vi "Handler - Fast Acq Loop.vi"(7 "Acquisition Start?":bool, 8 "error in (no error)":errorcluster, 9 "Acq Loop Data":T1, 10 "Loop Period":i64, 11 "Acquisition Period":i64) -> (0 "error out":errorcluster)   [LabVIEW 2018]
uses:
  Variables/Global - Data Globals.vi
  <vilib>/ptbypt/NI_PtbyPt.lvlib
  FPGA/Controls/DAQ Input Data.ctl
  Private Controls/FPGA Write Queue Data.ctl
  Outputs.lvlib
  Private Controls/Acquisition Loop Data.ctl
  FPGA/FPGA VI Reference.ctl
  <vilib>/Modbus/master/Modbus Master.lvclass
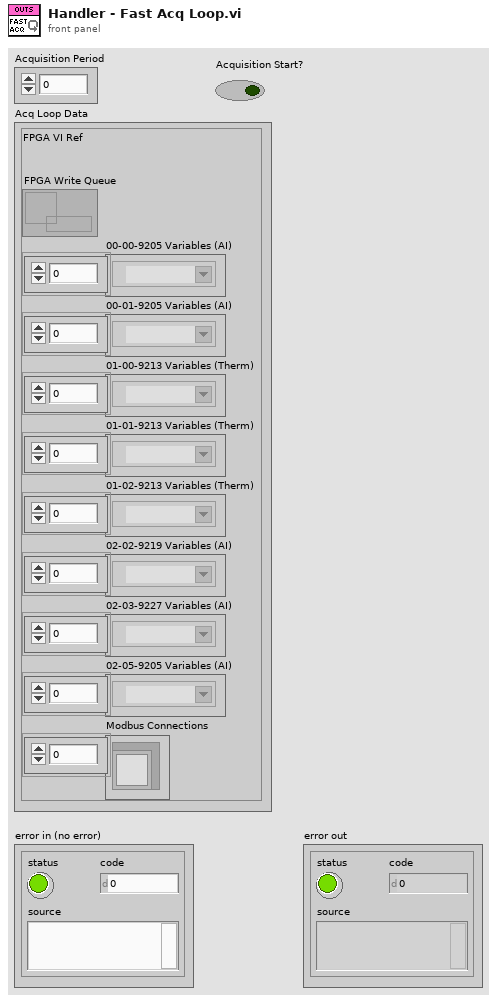
[diagram p1: front panel]
types:
  T1 = typedef "RT - Instrument IO.lvlib/Acquisition Loop Data.ctl" = cluster{"FPGA VI Ref":T2, "FPGA Write Queue":refnum<queue>, "00-00-9205 Variables (AI)":refnum<k21>[], "00-01-9205 Variables (AI)":refnum<k21>[], "01-00-9213 Variables (Therm)":refnum<k21>[], "01-01-9213 Variables (Therm)":refnum<k21>[], "01-02-9213 Variables (Therm)":refnum<k21>[], "02-02-9219 Variables (AI)":refnum<k21>[], "02-03-9227 Variables (AI)":refnum<k21>[], "02-05-9205 Variables (AI)":refnum<k21>[], "Modbus Connections":refnum<class "Modbus Master.lvclass">[]}
  T2 = typedef "FPGA VI Reference.ctl" = refnum<k20>
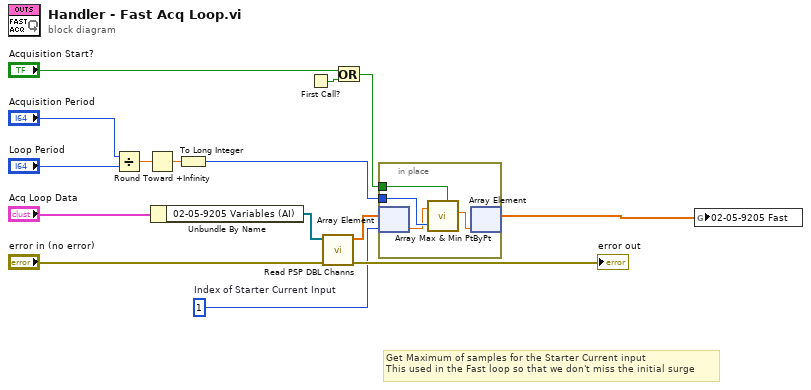
[diagram p0: block diagram]
diagram:
  w5 = 1  # Index of Starter Current Input
  # "Get Maximum of samples for the Starter Current input\nThis used in the Fast loop so that we don't miss the initial surge"
  n1 = Divide(x="Acquisition Period", y="Loop Period") -> (x/y=w13:dbl)
  n2 = Round Toward +Infinity(x=w13) -> (ceil(x): smallest int >= x=w12:dbl)
  n3 = Unbundle By Name("Acq Loop Data") -> ("02-05-9205 Variables (AI)"=w11:refnum<k21>[])
  n4 = To Long Integer(number=w12) -> (32bit integer=w7:i32)
  n5 = First Call?() -> (First Call?: T/F=w3:bool)
  n6 = call "Read PSP DBL Channs.vi"("error in (no error)"="error in (no error)", "PSP Variables in"=w11) -> ("error out"=→"error out":errorcluster, "Data out"=w6:dbl[])  [unwired: 8 in]
  n7 = Or(x="Acquisition Start?", y=w3) -> (x .or. y?=w1:bool)
  n8 = in-place {
    in-place-border: w7 -> [w19]
    in-place-border: w1 -> [w17]
    n9 = in-place-array #1(w6, w5) -> (w16:dbl)
    n10 = call <vilib>:"Array Max & Min PtByPt.vi"("input data point"=w16, "sample length"=w19, "initialize"=w17) -> ("max value"=w18:dbl)  [unwired: 4 out]
    n11 = in-place-array #1(w18) -> (w4:dbl[])  [unwired: 1 out]
  }
  n12 = global write "Global - Data Globals.vi" "02-05-9205 Fast"(w4) -> ()
